vi "convertCluster.vi"(10 "Data":T1={"cRIO Data"={"Time (ms)"=0.0, "24V Battery (V)"=0.0, "LowV Current (A)"=0.0, "Fiducial Sensor (V)"=0.0, "PV Pressure (psig)"=0.0, "Flow Sensor (V)"=0.0, "Temp Fairing (F)"=0.0, "Temp Reservoir (F)"=0.0, "HallEffect Right (in)"=0.0, "HallEffect Left (in)"=0.0, "PT Tank (psig)"=0.0, "PT Clamp Right (psig)"=0.0, "PT Clamp Left (psig)"=0.0, "PT Brake (psig)"=0.0, "PT Cooling (psig)"=0.0, "Displacement (ft)"=0.0, "Velocity (ft/s)"=0.0}, "IMU Data"={"x acceleration (g)"=0.0, "Pressure (psia)"=0.0, "Temperature (F)"=0.0}, "BMS Data"={"Max Cell Voltage (V)"=0.0, "Max Cell ID"=0.0, "Min Cell Voltage (V)"=0.0, "Min Cell ID"=0.0, "State of Charge (%)"=0.0, "Average Voltage (V)"=0.0, "Voltage Delta (V)"=0.0, "Pack Current (A)"=0.0, "Pack Voltage (V)"=0.0, "Max Resistance (Ohm)"=0.0, "Min Resistance (Ohm)"=0.0, "Average Resistance (Ohm)"=0.0, "Delta Resistance (Ohm)"=0.0, "Highest Temperature(F)"=0.0, "BmsStatus"={"isFault"=FALSE, "isolationMonitoring"=FALSE}}, "Motor Data"={"Velo (RPM)"=0.0, "MotorTemp(F)"=0.0, "CtrlTemp(F)"=0.0, "DcLinkVolt(V)"=0.0, "ErrorCode"=0.0, "motorStatus"={"isReady"=FALSE, "isOn"=FALSE, "isOperEn"=FALSE, "isFault"=FALSE, "isVoltEn"=FALSE, "targetReached"=FALSE, "isWarning"=FALSE}, "isAlive"=FALSE, "motorControllerState"=1}} {"Motor Data"."motorControllerState" items=["unknown"=1, "boot-up"=0, "stopped"=4, "operational"=5, "pre-operational"=127, "connection lost"=128]}) -> (2 "Array":dbl[](array[numeric]))   [LabVIEW 2017]
uses:
  DAQ/Master_DataControl.ctl
  DAQ/TypeDef_cRIOData.ctl
  IMU/TypeDef_IMUData.ctl
  CAN/TypeDef_BMSData.ctl
  CAN/TypeDef_BMS_Status.ctl
  CAN/MotorController/fixedMotorData.ctl
  CAN/MotorController/MotorStatus.ctl
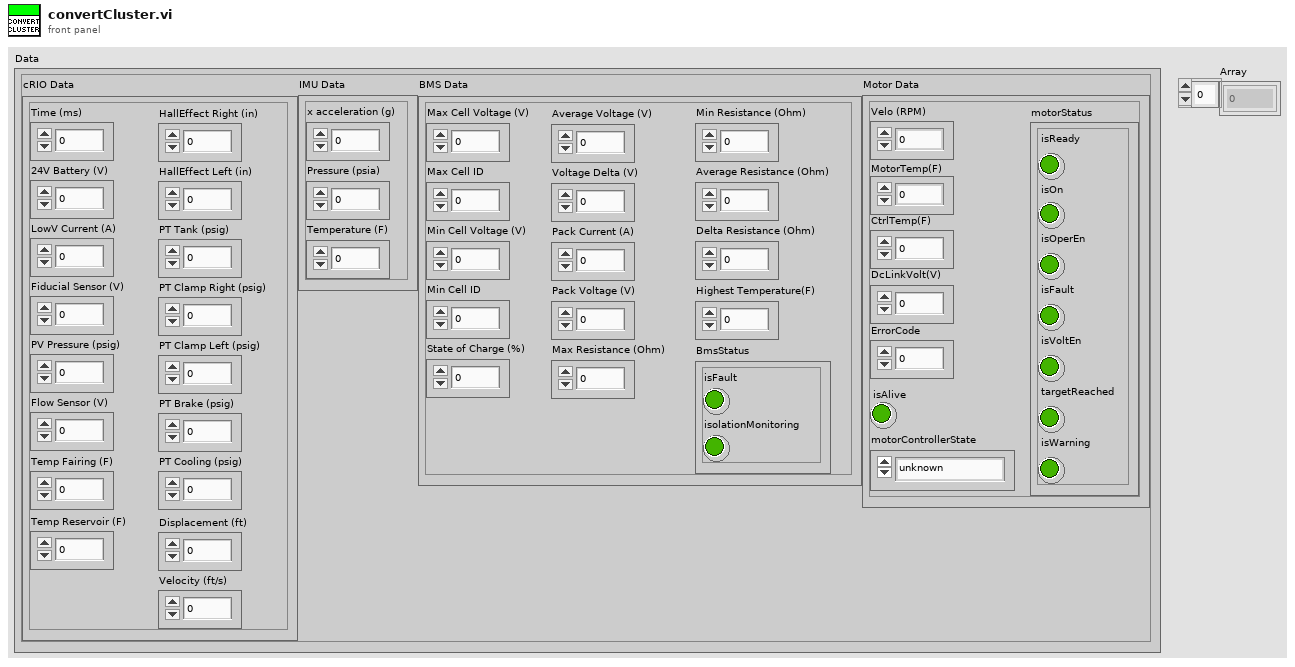
[diagram p1: front panel]
types:
  T1 = typedef "Master_DataControl.ctl" = cluster{"cRIO Data":T2, "IMU Data":T3, "BMS Data":T4, "Motor Data":T6}
  T2 = typedef "TypeDef_cRIOData.ctl" = cluster{"Time (ms)":dbl, "24V Battery (V)":dbl, "LowV Current (A)":dbl, "Fiducial Sensor (V)":dbl, "PV Pressure (psig)":dbl, "Flow Sensor (V)":dbl, "Temp Fairing (F)":dbl, "Temp Reservoir (F)":dbl, "HallEffect Right (in)":dbl, "HallEffect Left (in)":dbl, "PT Tank (psig)":dbl, "PT Clamp Right (psig)":dbl, "PT Clamp Left (psig)":dbl, "PT Brake (psig)":dbl, "PT Cooling (psig)":dbl, "Displacement (ft)":dbl, "Velocity (ft/s)":dbl}
  T3 = typedef "TypeDef_IMUData.ctl" = cluster{"x acceleration (g)":dbl, "Pressure (psia)":dbl, "Temperature (F)":dbl}
  T4 = typedef "TypeDef_BMSData.ctl" = cluster{"Max Cell Voltage (V)":dbl, "Max Cell ID":dbl, "Min Cell Voltage (V)":dbl, "Min Cell ID":dbl, "State of Charge (%)":dbl, "Average Voltage (V)":dbl, "Voltage Delta (V)":dbl, "Pack Current (A)":dbl, "Pack Voltage (V)":dbl, "Max Resistance (Ohm)":dbl, "Min Resistance (Ohm)":dbl, "Average Resistance (Ohm)":dbl, "Delta Resistance (Ohm)":dbl, "Highest Temperature(F)":dbl, "BmsStatus":T5}
  T5 = typedef "TypeDef_BMS_Status.ctl" = cluster{"isFault":bool, "isolationMonitoring":bool}
  T6 = typedef "fixedMotorData.ctl" = cluster{"Velo (RPM)":dbl, "MotorTemp(F)":dbl, "CtrlTemp(F)":dbl, "DcLinkVolt(V)":dbl, "ErrorCode":dbl, "motorStatus":T7, "isAlive":bool, "motorControllerState":u16}
  T7 = typedef "MotorStatus.ctl" = cluster{"isReady":bool, "isOn":bool, "isOperEn":bool, "isFault":bool, "isVoltEn":bool, "targetReached":bool, "isWarning":bool}
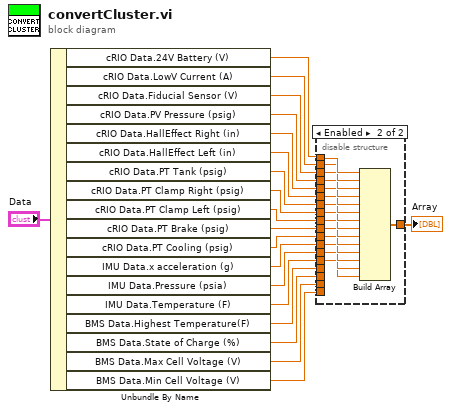
[diagram p0: block diagram]
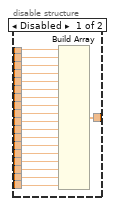
[diagram p2: hidden frame]
diagram:
  n1 = Unbundle By Name("Data") -> ("cRIO Data.24V Battery (V)"=w19:dbl, "cRIO Data.LowV Current (A)"=w18:dbl, "cRIO Data.Fiducial Sensor (V)"=w17:dbl, "cRIO Data.PV Pressure (psig)"=w16:dbl, "cRIO Data.HallEffect Right (in)"=w15:dbl, "cRIO Data.HallEffect Left (in)"=w14:dbl, "cRIO Data.PT Tank (psig)"=w13:dbl, "cRIO Data.PT Clamp Right (psig)"=w12:dbl, "cRIO Data.PT Clamp Left (psig)"=w11:dbl, "cRIO Data.PT Brake (psig)"=w10:dbl, "cRIO Data.PT Cooling (psig)"=w9:dbl, "IMU Data.x acceleration (g)"=w8:dbl, "IMU Data.Pressure (psia)"=w7:dbl, "IMU Data.Temperature (F)"=w5:dbl, "BMS Data.Highest Temperature(F)"=w4:dbl, "BMS Data.State of Charge (%)"=w3:dbl, "BMS Data.Max Cell Voltage (V)"=w2:dbl, "BMS Data.Min Cell Voltage (V)"=w1:dbl)
  n2 = disable-structure shown="Enabled" {
    disable-tunnel: w19 -> [w39 w54]
    disable-tunnel: w18 -> [w38 w53]
    disable-tunnel: w17 -> [w37 w52]
    disable-tunnel: w16 -> [w36 w51]
    disable-tunnel: w15 -> [w35 w50]
    disable-tunnel: w14 -> [w34 w49]
    disable-tunnel: w13 -> [w33 w48]
    disable-tunnel: w12 -> [w32 w47]
    disable-tunnel: w11 -> [w31 w46]
    disable-tunnel: w10 -> [w30 w45]
    disable-tunnel: w9 -> [w29 w44]
    disable-tunnel: w8 -> [w28 w43]
    disable-tunnel: w7 -> [w27 w42]
    disable-tunnel: [w26 w40] -> w6
    disable-tunnel: w5 -> [w25 w41]
    disable-tunnel: w4 -> [w24 _]
    disable-tunnel: w3 -> [w23 _]
    disable-tunnel: w2 -> [w22 _]
    disable-tunnel: w1 -> [w21 _]
    frame Disabled {
      n3 = Build Array(w39, w38, w37, w36, w35, w34, w33, w32, w31, w30, w29, w28, w27, w25, w24, w23, w22, w21) -> (w26:dbl[])
    }
    frame Enabled {
      n4 = Build Array(w54, w53, w52, w51, w50, w49, w48, w47, w46, w45, w44, w43, w42, w41) -> (w40:dbl[])
    }
  }
  "Array" <- w6
